vi "Untitled 1.vi"() -> ()   [LabVIEW 2015]
uses:
  Program Files (x86)/National Instruments/LabVIEW 2015/examples/robotics/Vision/Color Tracking/HueSlider.ctl
  <vilib>/userdefined/High Color/IMAQdx.ctl
  <vilib>/vision/driver/NI_Vision_Acquisition_Software.lvlib
panel:
  out "Input Image":T1(plugin-control)
  out "Processed Image":T1(plugin-control)
  in  "Stop (F)":bool caption="Stop"
  in  "Hue range":T2={"Min"=232, "Max"=21} scale=0.0..255.0
  in  "Select Color":u16(ring) items=["Red", "Green", "Custom"]
  in  "Loop Delay (ms)":u32(slide)=150 scale=0.0..250.0
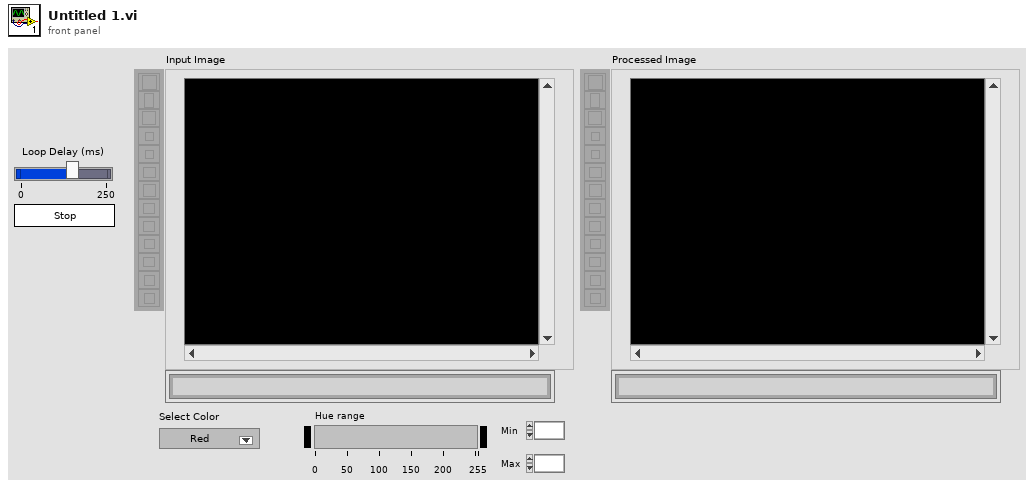
[diagram p1: front panel]
types:
  T1 = typedef "IMAQ Image.ctl" = refnum<image>
  T2 = typedef "HueSlider.ctl" = cluster{"Min":i32, "Max":i32}
  T3 = typedef "IMAQdx.ctl" = refnum<k21>
  T4 = typedef "IMAQ Circle" = cluster{"Center X":i32, "Center Y":i32, "Inner Radius":i32, "Outer Radius":i32, "Start Angle":dbl, "End Angle":dbl}
  T5 = enum8{"Enabled", "Disabled", "Disabled and Grayed Out"}
  T6 = cluster{"Center":cluster{"X":sgl, "Y":sgl}, "Radius":dbl}
  T7 = typedef "ROI Descriptor" = cluster{"Global Rectangle":i32[], "Contours":cluster{"ID":enum32{"External", "Internal"}, "Type":u32, "Coordinates":i32[]}[]}
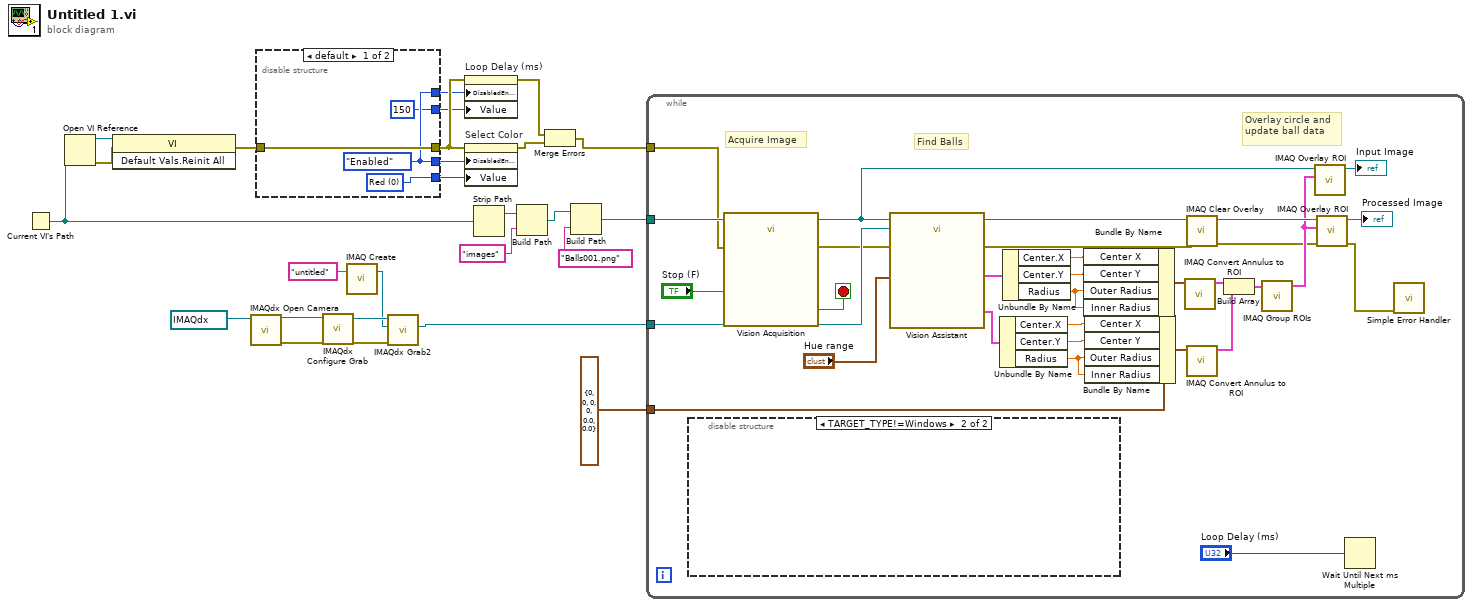
[diagram p0: block diagram]
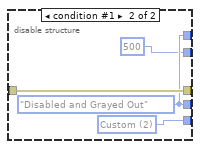
[diagram p2: hidden frame]
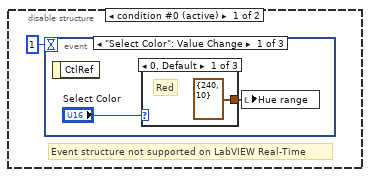
[diagram p3: hidden frame]
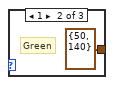
[diagram p4: hidden frame]
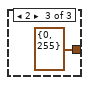
[diagram p5: hidden frame]
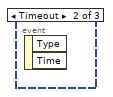
[diagram p6: hidden frame]
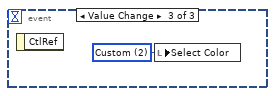
[diagram p7: hidden frame]
diagram:
  n1 = Current VI's Path() -> (path=w19:path)
  n2 = Open VI Reference(vi path=w19) -> (vi reference=w20:refnum<vi>, error out=w18:errorcluster)  [unwired: 5 in]
  n3 = invoke class="VI" method="Default Vals.Reinit All"(reference=w20, error in=w18) -> (error out=w15:errorcluster)  [unwired: 1 in, 2 out]
  n4 = call <vilib>:"IMAQdx Open Camera.vi"("Session In"=T3 "cam3") -> ("error out"=w6:errorcluster, "Session Out"=w7:T3)  [unwired: 9 in]
  n5 = disable-structure shown="default" {
    disable-tunnel: [w28 w32] -> w17
    disable-tunnel: [w30 w34] -> w16
    disable-tunnel: [w29 w33] -> w14
    disable-tunnel: w15 -> [w29 w33]
    disable-tunnel: [w28 w32] -> w10
    disable-tunnel: [u32 150 ("Loop Delay (ms)") u32 500 ("Loop Delay (ms)")] -> w9
    frame condition #0 (active) {
      w30 = u16 0 items=["Red", "Green", "Custom"] ("Select Color")
      w28 = T5."Enabled" ("Disabled")
    }
    frame condition #1 {
      w34 = u16 2 items=["Red", "Green", "Custom"] ("Select Color")
      w32 = T5."Disabled and Grayed Out" ("Disabled")
    }
  }
  n6 = call <vilib>:"IMAQdx Configure Grab.vi"("error in"=w6, "Session In"=w7) -> ("error out"=w4:errorcluster, "Session Out"=w5:T3)  [unwired: 8 in]
  n7 = call "IMAQ Create"("Image Name"="untitled") -> ("New Image"=w2:T1)  [unwired: 3 in, 2 out]
  n8 = call <vilib>:"IMAQdx Grab2.vi"("error in"=w4, "Image In"=w2, "Session In"=w5) -> ("Image Out"=w3:T1)  [unwired: 5 in, 3 out]
  n9 = property on="Loop Delay (ms)" class="Slide (strict)"(error in=w14, "DisabledEnum"=w10, "Value"=w9) -> (error out=w12:errorcluster)  [unwired: 1 in, 1 out]
  n10 = property on="Select Color" class="Ring (strict)"(error in=w14, "DisabledEnum"=w17, "Value"=w16) -> (error out=w13:errorcluster)  [unwired: 1 in, 1 out]
  n11 = Strip Path(path=w19) -> (stripped path=w25:path)  [unwired: 1 out]
  n12 = Build Path(base path=w25, name or relative path="images") -> (appended path=w23:path)
  n13 = Merge Errors(w12, w13) -> (w11:errorcluster)
  n14 = Build Path(base path=w23, name or relative path="Balls001.png") -> (appended path=w21:path)
  n15 = while {
    tunnel: w3 -> [w64]
    tunnel: T4 {"Center X"=0, "Center Y"=0, "Inner Radius"=0, "Outer Radius"=0, "Start Angle"=0.0, "End Angle"=0.0} ("Annulus") -> [w59]
    tunnel: w21 -> [w39]
    tunnel: w11 -> [w36]
    stop <- w65 stop-if-true
    # "Overlay circle and update ball data"
    # "Find Balls"
    # "Acquire Image"
    n16 = disable-structure shown="TARGET_TYPE!=Windows" {
      frame condition #0 (active) {
        # "Event structure not supported on LabVIEW Real-Time"
        n17 = event shown="[0] \"Select Color\": Value Change" {
          selector: _ -> [_ _ _]
          dyn-events: _ -> [_ _ _]
          timeout: 1 -> [_ _ _]
          event "Select Color": Value Change {
            n18 = event-data() -> ()  [unwired: 1 in, 1 out]
            n19 = case shown="0, Default" "Select Color" {
              tunnel: [cluster{"Lower value":i32, "Upper value":i32} {"Lower value"=240, "Upper value"=10} ("Red or Hue Range (Color Threshold)") cluster{"Lower value":i32, "Upper value":i32} {"Lower value"=50, "Upper value"=140} ("Red or Hue Range (Color Threshold)") cluster{"Lower value":i32, "Upper value":i32} {"Lower value"=0, "Upper value"=255} ("Red or Hue Range (Color Threshold)")] -> w67
              frame 0, Default {
                # "Red"
              }
              frame 1 {
                # "Green"
              }
              frame 2 {
              }
            }
            n20 = local write "Hue range"(w67) -> ()
          }
          event Timeout {
            n21 = event-data() -> ()  [unwired: 1 in, 2 out]
          }
          event Value Change {
            w72 = u16 2 items=["Red", "Green", "Custom"] ("Select Color")
            n22 = event-data() -> ()  [unwired: 1 in, 1 out]
            n23 = local write "Select Color"(w72) -> ()
          }
        }
      }
      frame condition #1 {
      }
    }
    n24 = call "Vision Acquisition"("Image Path"=w39, "Stop (F)"="Stop (F)", "error in"=w36) -> ("Image Out"=w51:T1, "Stopped"=w65:bool, "error out"=w63:errorcluster)  [unwired: 22 out]
    n25 = call "Vision Assistant"("Image In"=w51, "Image Dst"=w64, "Red or Hue Range (Color Threshold)"="Hue range", "error in"=w63) -> ("Image Out"=w46:T1, "Best Circle (Fit Circle Ball 1)"=w62:T6, "Best Circle (Fit Circle Ball 2)"=w49:T6, "error out"=w42:errorcluster)  [unwired: 20 out]
    n26 = Unbundle By Name(w49) -> ("Center.X"=w58:sgl, "Center.Y"=w57:sgl, "Radius"=w48:dbl)
    n27 = Unbundle By Name(w62) -> ("Center.X"=w61:sgl, "Center.Y"=w60:sgl, "Radius"=w47:dbl)
    n28 = Bundle By Name(cluster=w59, "Center X"=w61, "Center Y"=w60, "Outer Radius"=w47, "Inner Radius"=w47) -> (w56:T4)
    n29 = Bundle By Name(cluster=w59, "Center X"=w58, "Center Y"=w57, "Outer Radius"=w48, "Inner Radius"=w48) -> (w55:T4)
    n30 = call "IMAQ Convert Annulus to ROI"("Annulus"=w56) -> ("ROI Descriptor"=w54:T7)  [unwired: 1 in, 8 out]
    n31 = call "IMAQ Clear Overlay"("error in (no error)"=w42, "Image"=w46) -> ("error out"=w41:errorcluster, "Image Out"=w45:T1)  [unwired: 1 in, 7 out]
    n32 = call "IMAQ Convert Annulus to ROI"("Annulus"=w55) -> ("ROI Descriptor"=w53:T7)  [unwired: 1 in, 8 out]
    n33 = Build Array(w54, w53) -> (w52:T7[])
    n34 = call "IMAQ Group ROIs"("ROI Descriptors"=w52) -> ("ROI Descriptor out"=w43:T7)  [unwired: 1 in, 3 out]
    n35 = call "IMAQ Overlay ROI"("ROI Descriptor"=w43, "Image"=w51) -> ("Image Out"=→"Input Image":T1)  [unwired: 4 in, 5 out]
    n36 = call "IMAQ Overlay ROI"("error in (no error)"=w41, "ROI Descriptor"=w43, "Image"=w45) -> ("error out"=w38:errorcluster, "Image Out"=→"Processed Image":T1)  [unwired: 3 in, 4 out]
    n37 = Wait Until Next ms Multiple(millisecond multiple="Loop Delay (ms)") -> ()  [unwired: 1 out]
    n38 = call <vilib>:"Simple Error Handler.vi"("error in (no error)"=w38) -> ()  [unwired: 1 in, 8 out]
  }
